vi "VCM_Open_Queue.vi"(8 "error in (no error)":errorcluster) -> (0 "error out":errorcluster, 2 "queue out":refnum<queue>)   [LabVIEW 2019]
uses:
  Mischer/VCM-Control.ctl
  Global/Global Variables/Queues_global.vi
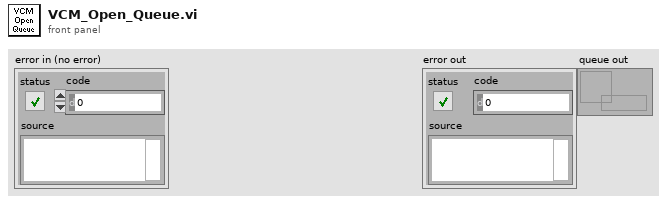
[diagram p1: front panel]
types:
  T1 = typedef "VCM-Control.ctl" = cluster{"Steps":dbl, "Amplitude SET":dbl, "Frequenz":dbl, "A max":dbl, "Update VCM":bool}
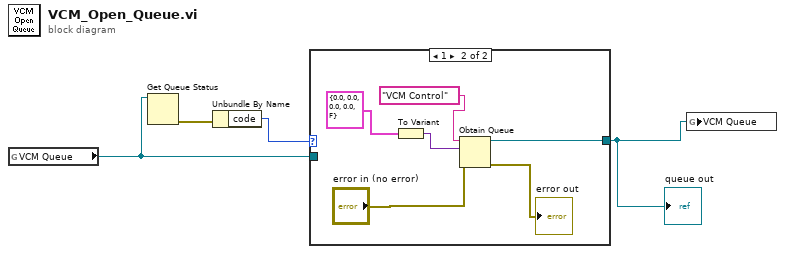
[diagram p0: block diagram]
diagram:
  n1 = global read "Queues_global.vi" "VCM Queue"() -> (w2:refnum<queue>)
  n2 = Get Queue Status(queue=w2) -> (error out=w4:errorcluster)  [unwired: 2 in, 7 out]
  n3 = Unbundle By Name(w4) -> ("code"=w3:i32)
  n4 = case shown="1" w3 {
    tunnel: w2 -> [w5 _]
    tunnel: [w5 w8] -> w1
    frame 0, Default {
    }
    frame 1 {
      n5 = To Variant(anything=T1 {"Steps"=0.0, "Amplitude SET"=0.0, "Frequenz"=0.0, "A max"=0.0, "Update VCM"=FALSE} ("VCM Control")) -> (Variant=w6:variant)
      n6 = Obtain Queue(name (unnamed)="VCM Control", element data type=w6, error in (no error)="error in (no error)") -> (queue out=w8:refnum<queue>, error out=→"error out":errorcluster)  [unwired: 2 in, 1 out]
    }
  }
  "queue out" <- w1
  n7 = global write "Queues_global.vi" "VCM Queue"(w1) -> ()
